vi "ConnectionWriteData.vi"(8 "error in (no error)":errorcluster, 10 "DataToSend":refnum<class "DataToSend.lvclass">, 11 "TcpServer in":refnum<class "TcpServer.lvclass">) -> (0 "error out":errorcluster, 3 "TcpServer out":refnum<class "TcpServer.lvclass">)   [LabVIEW 2022 SP3, in "TcpServer.lvlib" / "TcpServer.lvclass"]
uses:
  TcpServer.lvclass
  C:/Users/jakub/repos/gh/sw4sys/lv-tcp-server-sample/LoggingActor/Source/LoggingActor/LoggingActor/LoggingActor.lvclass
  DataToSend/DataToSend.lvclass
  TcpServer.lvclass/TcpServer.ctl
  LoggingActor/Source/LoggingActor/LoggingActor/LoggingActor.lvclass/LoggingActor.ctl
  DataToSend/DataToSend.lvclass/DataToSend.ctl
  Connection/Connection Messages/WriteData Msg/WriteData Msg.lvclass/WriteData Msg.ctl
  <vilib>/ActorFramework/Message Enqueuer/Message Enqueuer.lvclass/Message Enqueuer.ctl
  DataToSend/Read Refnum.vi
  DataToSend/Read Data.vi
  LoggingActor/Source/LoggingActor/LoggingActor/Read Logger.vi
  <vilib>/ActorFramework/Message Enqueuer/Enqueue.vi
  Connection/Connection Messages/WriteData Msg/WriteData Msg.lvclass
  C:/Program Files (x86)/National Instruments/LabVIEW 2022/vi.lib/ActorFramework/Message/Message.lvclass
  <vilib>/ActorFramework/Message Priority Queue/Priority Enqueue.vi
  Logger/Source/Logger/Logger.lvclass
  StringUtils/Source/StringUtils/StringUtils.lvlib
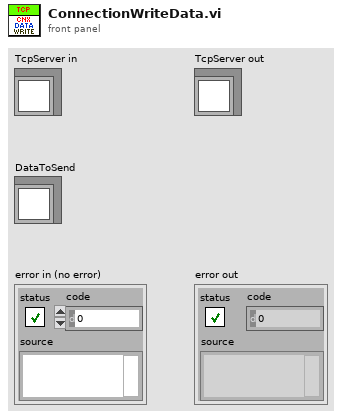
[diagram p1: front panel]
types:
  T1 = map{u64, refnum<class "Message Enqueuer.lvclass">}
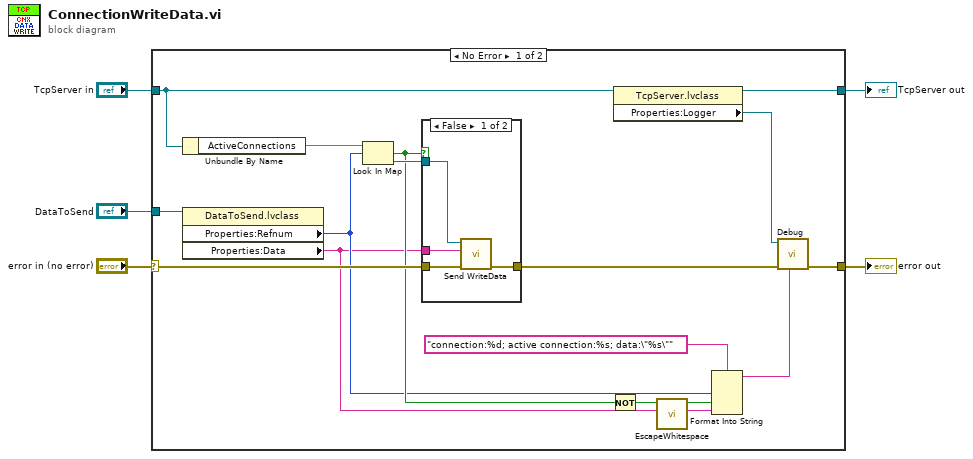
[diagram p0: block diagram]
diagram:
  n1 = case shown="No Error" "error in (no error)" {
    selector: "error in (no error)" -> [w21 w28]
    tunnel: [w15 w28] -> w4
    tunnel: [w8 w27] -> w2
    tunnel: "TcpServer in" -> [w20 w27]
    tunnel: "DataToSend" -> [w18 _]
    frame No Error {
      n2 = Unbundle By Name(w20) -> ("ActiveConnections"=w19:T1)
      n3 = property class="DataToSend.lvclass"(reference=w18) -> ("Properties:Refnum"=w12:u64, "Properties:Data"=w11:string)  [unwired: 1 in, 2 out]
      n4 = Look In Map(map=w19, key=w12) -> (key not found?=w13:bool, value=w16:refnum<class "Message Enqueuer.lvclass">)  [unwired: 1 in]
      n5 = case shown="False" w13 {
        tunnel: w21 -> [w25 w26]
        tunnel: [w24 w26] -> w17
        tunnel: w16 -> [w23 _]
        tunnel: w11 -> [w22 _]
        frame False {
          n6 = call "Send WriteData.vi"("error in (no error)"=w25, "Data"=w22, "Message Enqueuer"=w23) -> ("error out"=w24:errorcluster)  [unwired: 7 in, 1 out]
        }
        frame True {
        }
      }
      n7 = Not(x=w13) -> (.not. x?=w6:bool)
      n8 = property class="TcpServer.lvclass"(reference=w20) -> (reference out=w8:refnum<class "TcpServer.lvclass">, "Properties:Logger"=w7:refnum<class "Logger.lvclass">)  [unwired: 1 in, 1 out]
      n9 = call "EscapeWhitespace.vi"("InputString"=w11) -> ("EscapedWhitespace"=w10:string)  [unwired: 10 in]
      n10 = Format Into String(format string="connection:%d; active connection:%s; data:\"%s\"", w12, w6, w10) -> (resulting string=w9:string)  [unwired: 2 in, 1 out]
      n11 = call-dynamic "Debug.vi"("Message"=w9, "error in (no error)"=w17, "Logger in"=w7) -> ("error out"=w15:errorcluster)  [unwired: 5 in, 1 out]
    }
    frame Error {
    }
  }
  "error out" <- w4
  "TcpServer out" <- w2
